vi "Set_Number_of_DL_Antennas.vi"(8 "error in (no error)":errorcluster, 9 "No of DL antennas Value":i32=1, 10 "Cellular Technology":T1, 11 "Base Station":T2) -> (0 "error out":errorcluster, 3 "Output String":string)   [LabVIEW 2021]
uses:
  Controls/Base_Station_Emulator.ctl
  Controls/Cellular_Technology.ctl
  Controls/TCP_FGV.ctl
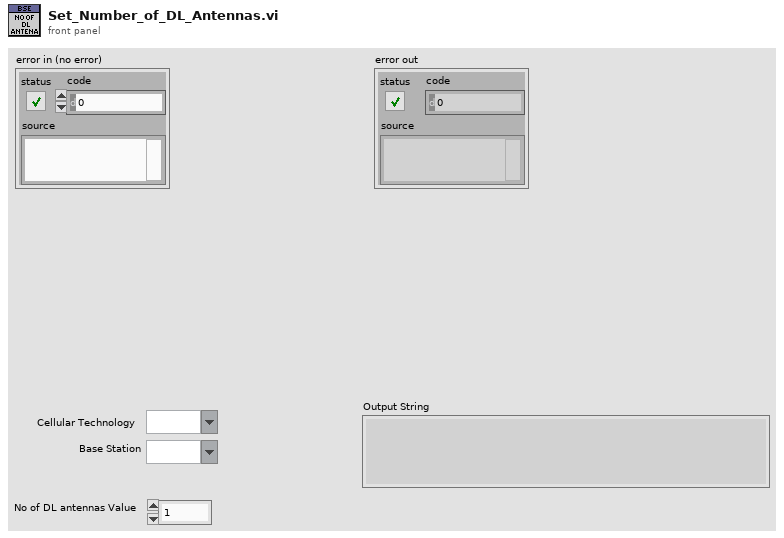
[diagram p1: front panel]
types:
  T1 = typedef "Cellular_Technology.ctl" = string
  T2 = typedef "Base_Station_Emulator.ctl" = string
  T3 = typedef "TCP_FGV.ctl" = enum16{"Open", "Read", "Write", "Close"}
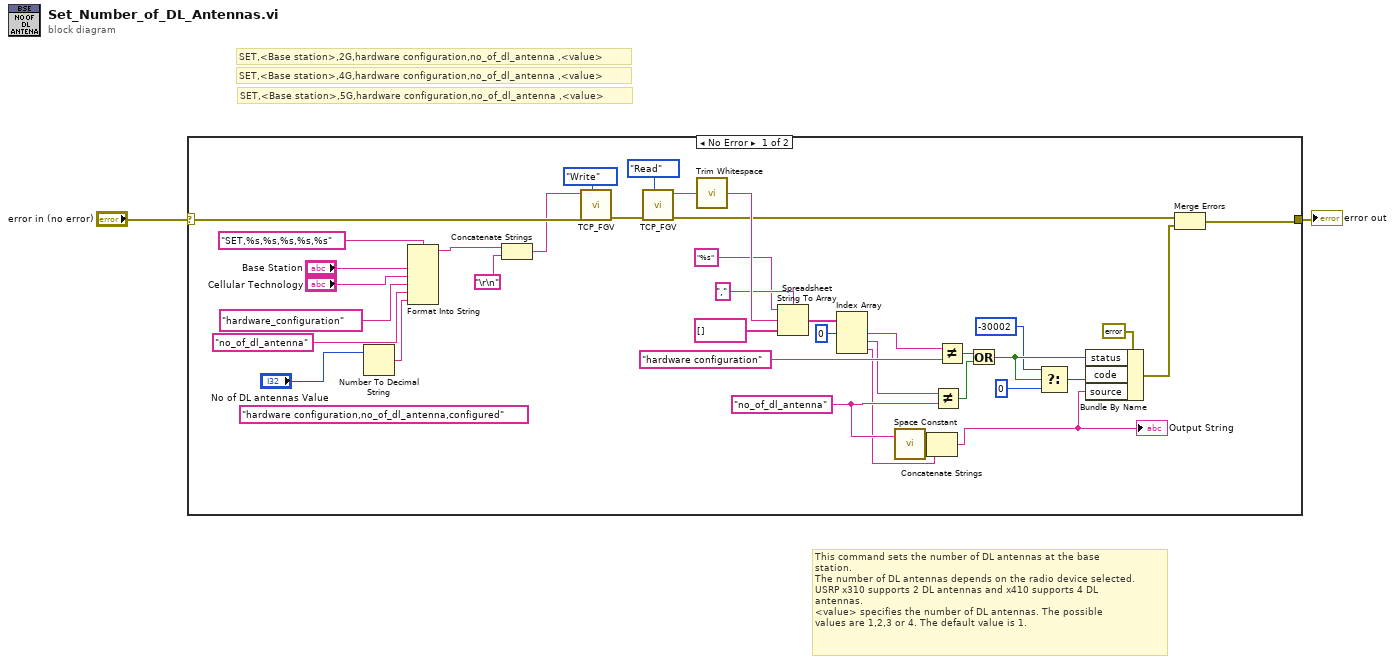
[diagram p0: block diagram]
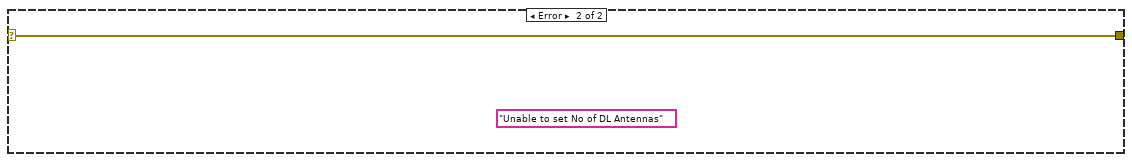
[diagram p2: hidden frame]
diagram:
  # "This command sets the number of DL antennas at the base \nstation. \nThe number of DL antennas depends on the radio device selected. \nUSRP x310 supports 2 DL antennas and x410 supports 4 DL \nantennas.  \n<value> specifies the number of DL antennas. The possible \nvalues are 1,2,3 or 4. The default value is 1."
  # "SET,<Base station>,5G,hardware configuration,no_of_dl_antenna ,<value>"
  # "SET,<Base station>,4G,hardware configuration,no_of_dl_antenna ,<value>"
  # "SET,<Base station>,2G,hardware configuration,no_of_dl_antenna ,<value>"
  n1 = case shown="No Error" "error in (no error)" {
    selector: "error in (no error)" -> [w38 w41]
    tunnel: [w16 w41] -> w1
    frame No Error {
      (unwired) "hardware configuration,no_of_dl_antenna,configured" ("format string")
      w12 = "no_of_dl_antenna"
      n2 = Number To Decimal String(number="No of DL antennas Value") -> (decimal integer string=w4:string)  [unwired: 1 in]
      n3 = Format Into String(format string="SET,%s,%s,%s,%s,%s", "Base Station", "Cellular Technology", "hardware_configuration", "no_of_dl_antenna", w4) -> (resulting string=w6:string)  [unwired: 2 in, 1 out]
      n4 = Concatenate Strings(w6, "\r\n") -> (w5:string)
      n5 = call "TCP_FGV.vi"("Command"=w5, "error in (no error)"=w38, "Operation"=TCP_FGV."Write") -> ("error out"=w17:errorcluster)  [unwired: 6 in, 1 out]
      n6 = call "TCP_FGV.vi"("error in (no error)"=w17, "Operation"=TCP_FGV."Read") -> ("Data Out"=w14:string, "error out"=w19:errorcluster)  [unwired: 7 in]
      n7 = call <vilib>:"Trim Whitespace.vi"("string"=w14) -> ("trimmed string"=w30:string)  [unwired: 1 in]
      n8 = Spreadsheet String To Array(delimiter (Tab)=",", format string="%s", spreadsheet string=w30, array type (2D Dbl)=string[] []) -> (array=w34:string[])
      n9 = Index Array(array=w34, index #1=0 ("index")) -> (element #1=w33:string, element #2=w15:string, element #3=w11:string)  [unwired: 2 in]
      n10 = call <vilib>:"Space Constant.vi"() -> ("String"=w13:string)
      n11 = Concatenate Strings(w12, w13, w11) -> (w10:string)
      "Output String" <- w10
      n12 = Not Equal?(x=w15, y=w12) -> (x != y?=w31:bool)
      n13 = Not Equal?(x=w33, y="hardware configuration" ("format string")) -> (x != y?=w32:bool)
      n14 = Or(x=w32, y=w31) -> (x .or. y?=w29:bool)
      n15 = Select(t=-30002 ("code"), s=w29, f=0 ("code")) -> (s? t:f=w28:i32)
      n16 = Bundle By Name(cluster=errorcluster {"status"=FALSE, "code"=0, "source"=""} ("error constant"), "status"=w29, "code"=w28, "source"=w10) -> (w18:errorcluster)
      n17 = Merge Errors(w19, w18) -> (w16:errorcluster)
    }
    frame Error {
      (unwired) "Unable to set No of DL Antennas" ("source")
    }
  }
  "error out" <- w1
